vi "Main.vi"() -> ()   [LabVIEW 2018, in "Command Pattern Demo.lvclass"]
uses:
  Command Pattern Demo.lvclass
  Stock Class/Stock.lvclass
  BuyStock Class/BuyStock.lvclass
  C:/Users/fflores/Documents/LabVIEW-Open-Projects/LabIVEW OOP Design Patterns/Command Pattern/Order Class/Order.lvclass
  SellStock Class/SellStock.lvclass
  Broker Class/Broker.lvclass
  ConsoleOut/Print Options.ctl
panel:
  out "error out":errorcluster
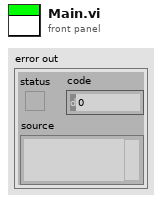
[diagram p1: front panel]
types:
  T1 = typedef "Print Options.ctl" = enum16{"Create", "Get Reference", "Print", "Print Header", "Close"}
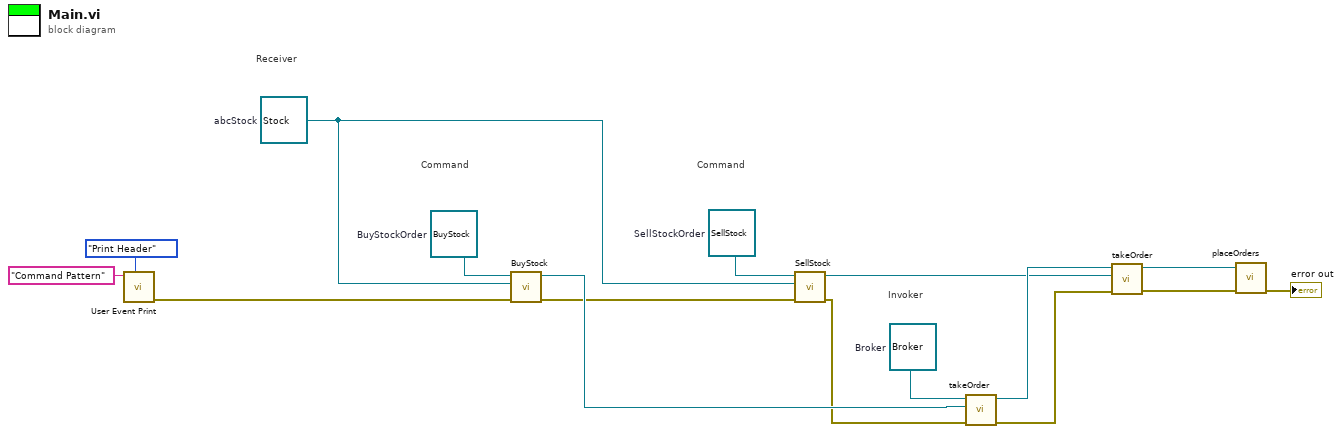
[diagram p0: block diagram]
diagram:
  w11 = refnum<class "Broker.lvclass"> refnum  # Broker
  w16 = refnum<class "SellStock.lvclass"> refnum  # SellStockOrder
  w15 = refnum<class "BuyStock.lvclass"> refnum  # BuyStockOrder
  w14 = refnum<class "Stock.lvclass"> refnum  # abcStock
  # "Invoker"
  # "Command"
  # "Command"
  # "Receiver"
  n1 = call "User Event Print.vi"("Options"=Print_Options."Print Header", "String to Print"="Command Pattern") -> ("error out"=w2:errorcluster)  [unwired: 8 in, 1 out]
  n2 = call "BuyStock.vi"("error in (no error)"=w2, "Stock.lvclass"=w14, "BuyStock in"=w15) -> ("error out"=w8:errorcluster, "BuyStock out"=w10:refnum<class "BuyStock.lvclass">)  [unwired: 7 in]
  n3 = call "SellStock.vi"("error in (no error)"=w8, "Stock.lvclass"=w14, "SellStock in"=w16) -> ("error out"=w7:errorcluster, "SellStock out"=w9:refnum<class "SellStock.lvclass">)  [unwired: 7 in]
  n4 = call "takeOrder.vi"("error in (no error)"=w7, "Order.lvclass"=w10, "Broker in"=w11) -> ("error out"=w12:errorcluster, "Broker out"=w13:refnum<class "Broker.lvclass">)  [unwired: 7 in]
  n5 = call "takeOrder.vi"("error in (no error)"=w12, "Order.lvclass"=w9, "Broker in"=w13) -> ("error out"=w5:errorcluster, "Broker out"=w6:refnum<class "Broker.lvclass">)  [unwired: 7 in]
  n6 = call "placeOrders.vi"("error in (no error)"=w5, "Broker in"=w6) -> ("error out"=→"error out":errorcluster)  [unwired: 8 in, 1 out]
